vi "Test Single Queue Regime.vi"(7 "Scan Status in":enum16{"Start", "Continue Scan", "Finish Scan"}(ring), 8 "Error in":errorcluster, 11 "Init?":bool=TRUE) -> (0 "Error Out":errorcluster)   [LabVIEW 2018]
uses:
  SerialSectOCT/SerialSectOCT/Software/General/Controls/QueueNames.ctl
  SerialSectOCT/SerialSectOCT/Software/General/Controls/MessagePacket.ctl
  SerialSectOCT/SerialSectOCT/Software/General/Controls/Queue Manager Actions.ctl
panel:
  in  "Channel":u32(ring)=1 items=["A"=1, "B"=2, "A + B"=3, "C"=4, "A + C"=5, "A + B"=6, "D"=8, "A + D"=9, "B + D"=10, "C + D"=12, "A + B + C + D"=15]
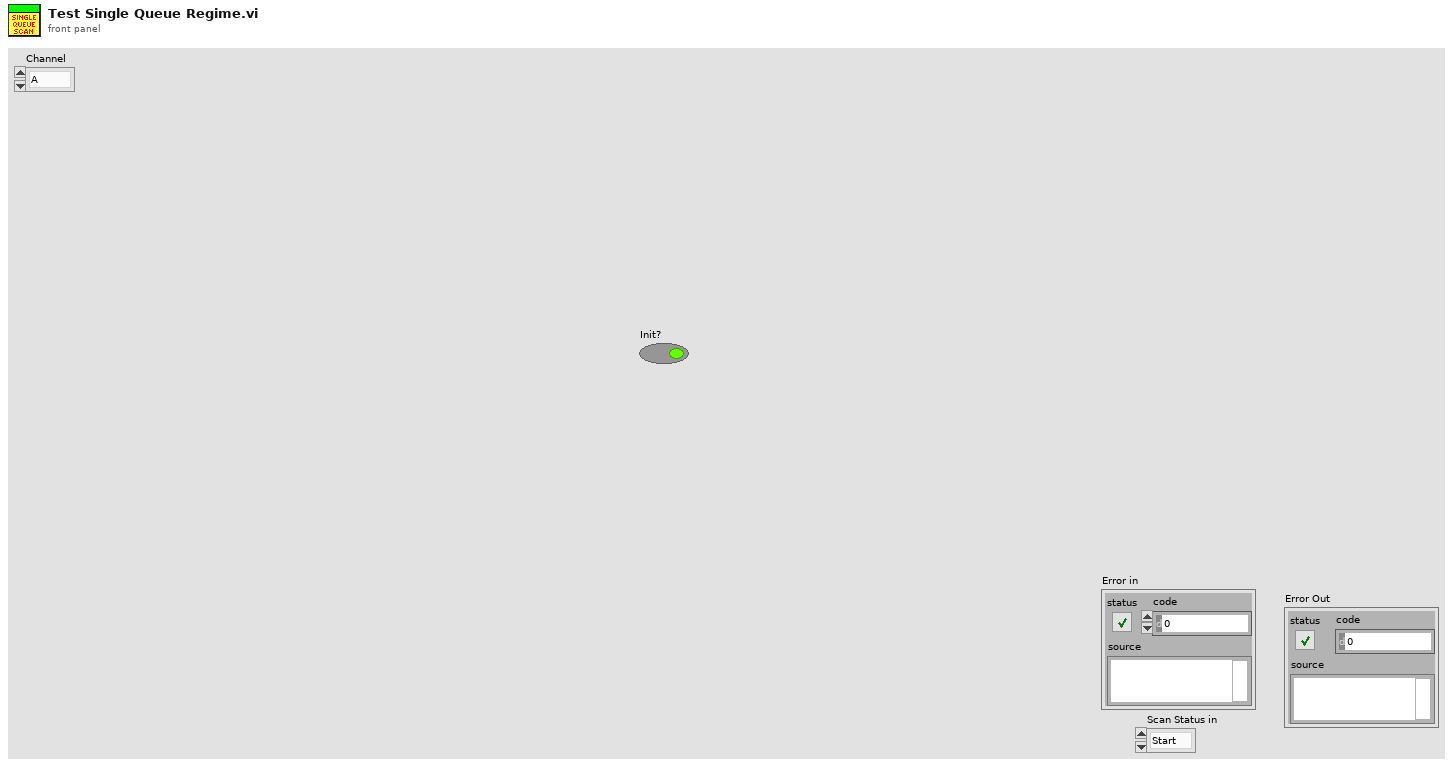
[diagram p1: front panel]
types:
  T1 = typedef "Queue Manager Actions.ctl" = enum16{"Init", "Enqueue", "Enqueue All", "Preview Queue", "Dequeue", "Get Status", "Flush Queue", "Flush All Queues", "Release All Queues", "Release Queue", "Enqueue at Opposite End"}
  T2 = typedef "MessagePacket.ctl" = cluster{"Message":string, "Parameter":variant}
  T3 = typedef "QueueNames.ctl" = enum16{"Main GUI", "Main Scan Processor", "Main Processing", "Main Saving", "Main Display", "Main Table Stage GUI", "Main Table Stage Proc.", "Scan Engine", "Vibratome GUI", "Vibratome Processor", "Slice Engine"}
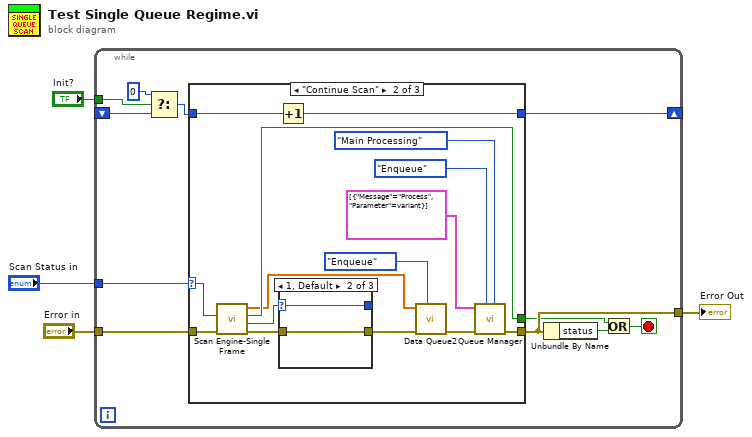
[diagram p0: block diagram]
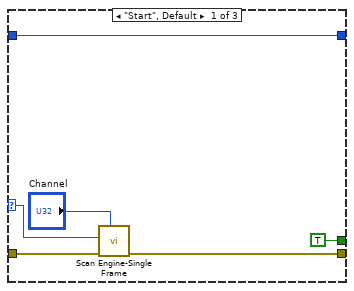
[diagram p2: hidden frame]
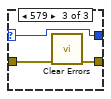
[diagram p4: hidden frame]
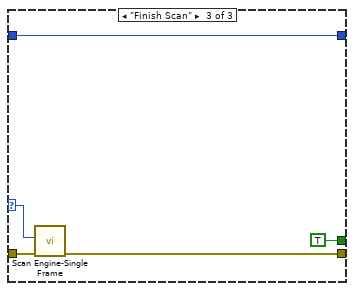
[diagram p5: hidden frame]
diagram:
  n1 = while {
    tunnel: "Error in" -> [w13]
    tunnel: "Scan Status in" -> [w15]
    tunnel: [w12] -> w2
    shift-right: [w14] -> _
    shift-left: _ -> [w7]
    tunnel: "Init?" -> [w5]
    stop <- w9 stop-if-true
    n2 = Select(t=u32 0, s=w5, f=w7) -> (s? t:f=w6:u32)
    n3 = case shown="\"Continue Scan\"" w15 {
      selector: w15 -> [w20 w35 w48]
      tunnel: w13 -> [w21 w36 w47]
      tunnel: [w18 w33 w44] -> w12
      tunnel: [TRUE w34 TRUE ("task done?")] -> w10
      tunnel: w6 -> [w16 w26 w45]
      tunnel: [w16 w25 w45] -> w14
      frame "Start", Default {
        n4 = call "Scan Engine-Single Frame.vi"("Channel"="Channel", "Error in"=w21, "Scan Status"=w20) -> ("Error Out"=w18:errorcluster)  [unwired: 5 in, 3 out]
      }
      frame "Continue Scan" {
        n5 = call "Scan Engine-Single Frame.vi"("Error in"=w36, "Scan Status"=w35) -> ("Error Out"=w24:errorcluster, "Return Code"=w22:u32, "task done?"=w34:bool, "data out"=w27:sgl[])  [unwired: 6 in]
        n6 = Increment(x=w26) -> (x+1=w25:u32)
        n7 = case shown="1, Default" w22 {
          selector: w22 -> [w38 w39 w41]
          tunnel: w24 -> [w37 w40 w43]
          tunnel: [w37 w40 w42] -> w23
          tunnel: [w38 w39 w41] -> _
          frame 0 {
          }
          frame 1, Default {
          }
          frame 579 {
            n8 = call <vilib>:"Clear Errors.vi"("error in (no error)"=w43) -> ("error out"=w42:errorcluster)  [unwired: 5 in, 1 out]
          }
        }
        n9 = call "Data Queue2.vi"("Action"=Queue_Manager_Actions."Enqueue", "error in (no error)"=w23, "data in"=w27) -> ("error out"=w28:errorcluster)  [unwired: 5 in, 3 out]
        n10 = call "Queue Manager.vi"("Queue Name"=QueueNames."Main Processing", "Action"=Queue_Manager_Actions."Enqueue", "Error In"=w28, "Message Packet Array"=T2[] [{"Message"="Process", "Parameter"=variant}]) -> ("Error Out"=w33:errorcluster)  [unwired: 3 in, 4 out]
      }
      frame "Finish Scan" {
        n11 = call "Scan Engine-Single Frame.vi"("Error in"=w47, "Scan Status"=w48) -> ("Error Out"=w44:errorcluster)  [unwired: 6 in, 3 out]
      }
    }
    n12 = Unbundle By Name(w12) -> ("status"=w11:bool)
    n13 = Or(x=w10, y=w11) -> (x .or. y?=w9:bool)
  }
  "Error Out" <- w2
